vi "Find Tunnels.vi"(11 "MultiDiagramStructure in":refnum<class "Structure.lvclass">) -> (2 "Tunnel Array":T1[](array[typedef]), 3 "Tunnels":map{string, T1}(c390))   [LabVIEW 2025]
uses:
  Classes/Node/Structure/Structure.lvclass
  Controls/Tunnel.ctl
  Controls/Terminal.ctl
  Classes/Node/Node.lvclass/Node.ctl
  <vilib>/regexp/Match Regular Expression.xnode
  Classes/Node/Node.lvclass
panel:
  out "Names":string[](array[string])
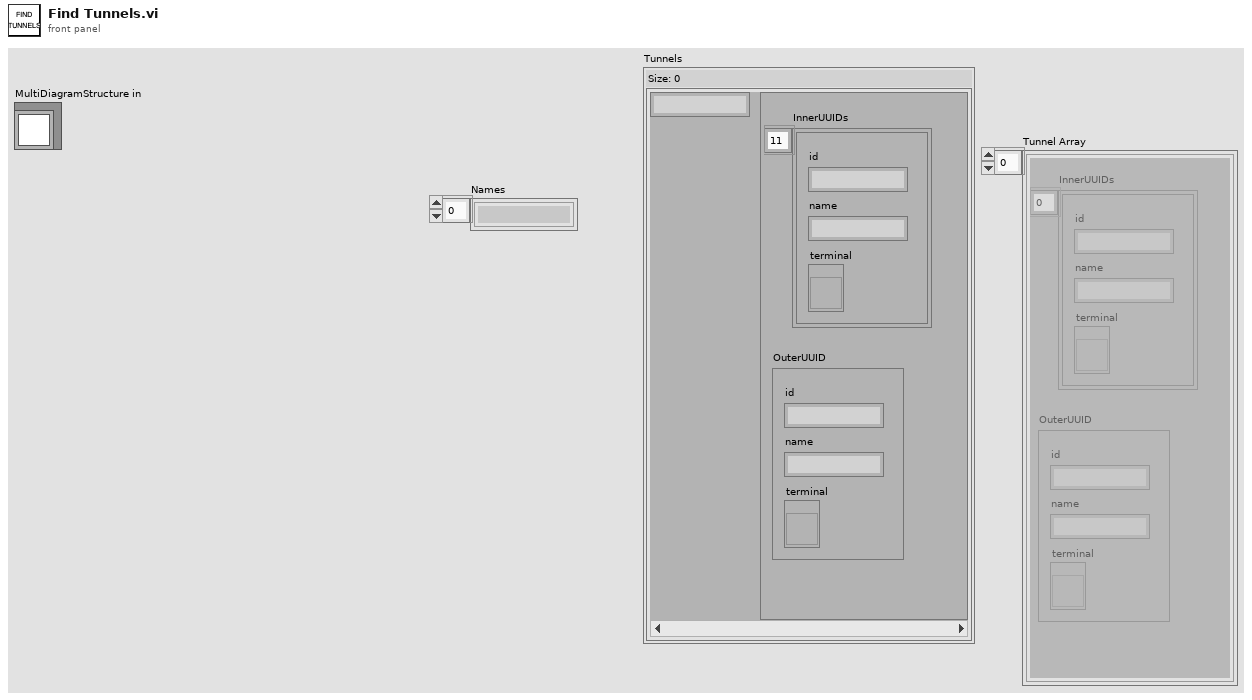
[diagram p1: front panel]
types:
  T1 = typedef "Tunnel.ctl" = cluster{"OuterUUID":T2, "InnerUUIDs":T2[]}
  T2 = typedef "Terminal.ctl" = cluster{"id":string, "name":string, "terminal":refnum<vi>}
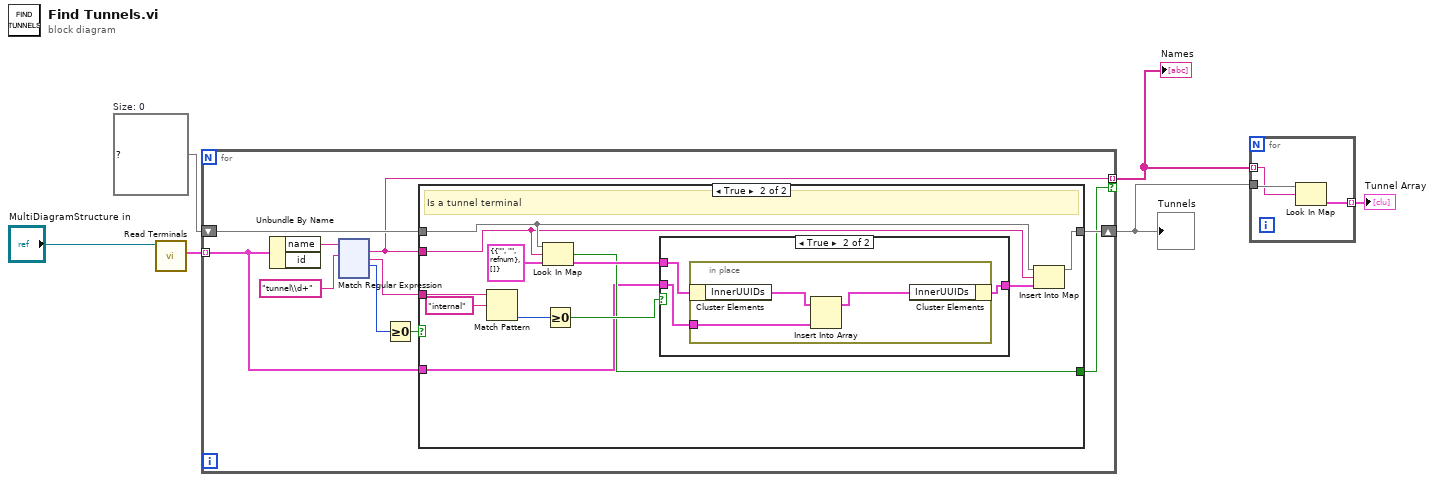
[diagram p0: block diagram]
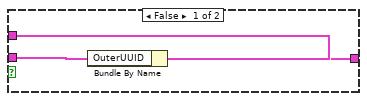
[diagram p3: hidden frame]
diagram:
  w6 = map{string, T1} {}  # Size: 0
  n1 = call "Read Terminals.vi"("Node in"="MultiDiagramStructure in") -> ("Terminals"=w4:T2[])  [unwired: 8 in, 2 out]
  n2 = for {
    tunnel: w4 -> [w7] mode=indexing
    shift-right: [w10] -> w2
    shift-left: w6 -> [w12]
    tunnel: [w9] -> w3 mode=indexing if=w8
    n3 = Unbundle By Name(w7) -> ("name"=w16:string)  [unwired: 1 out]
    n4 = xnode "Match Regular Expression"("input string"=w16, "regular expression"="tunnel\\d+") -> ("whole match"=w9:string, "after match"=w11:string, "offset past match"=w14:i32)  [unwired: 4 in, 2 out]
    n5 = Greater Or Equal To 0?(x=w14) -> (x >= 0?=w13:bool)
    n6 = case shown="True" w13 {
      selector: w13 -> [w17 _]
      tunnel: w12 -> [w18 w24]
      tunnel: w9 -> [_ w22]
      tunnel: w11 -> [_ w28]
      tunnel: [w18 w21] -> w10
      tunnel: [w17 w20] -> w8
      tunnel: w7 -> [_ w19]
      frame False {
        # "not a tunnel terminal"
      }
      frame True {
        # "Is a tunnel terminal"
        n7 = Match Pattern(string=w28, regular expression="internal") -> (offset past match=w26:i32)  [unwired: 1 in, 3 out]
        n8 = Look In Map(map=w24, key=w22, default value=T1 {"OuterUUID"={"id"="", "name"="", "terminal"=refnum}, "InnerUUIDs"=[]}) -> (key not found?=w20:bool, value=w29:T1)
        n9 = Greater Or Equal To 0?(x=w26) -> (x >= 0?=w25:bool)
        n10 = case shown="True" w25 {
          tunnel: w29 -> [w33 w36]
          tunnel: w19 -> [w32 w34]
          tunnel: [w31 w35] -> w23
          frame False {
            n11 = Bundle By Name(cluster=w33, "OuterUUID"=w32) -> (w31:T1)
          }
          frame True {
            n12 = in-place {
              in-place-border: w34 -> [w37]
              n13 = in-place-cluster #1(w36) -> ("InnerUUIDs"=w39:T2[])
              n14 = Insert Into Array(array=w39, new element=w37) -> (w38:T2[])  [unwired: 1 in]
              n15 = in-place-cluster #1("InnerUUIDs"=w38) -> (w35:T1)
            }
          }
        }
        n16 = Insert Into Map(map in=w24, key=w22, value=w23) -> (map out=w21:map{string, T1})  [unwired: 2 out]
      }
    }
  }
  "Tunnels" <- w2
  "Names" <- w3
  n17 = for {
    tunnel: w3 -> [w158] mode=indexing
    tunnel: w2 -> [w159]
    tunnel: [w157] -> w1 mode=indexing
    n18 = Look In Map(map=w159, key=w158) -> (value=w157:T1)  [unwired: 1 in, 1 out]
  }
  "Tunnel Array" <- w1
